vi "Get XPath Text.vi"(8 "error in (no error)":errorcluster, 10 "XPath Expression":string, 11 "DOM document in":refnum<k20>) -> (0 "error out":errorcluster, 1 "Found?":bool, 2 "Node Text":string, 3 "DOM document out":refnum<k20>)   [LabVIEW 2016, in "SLL File IO.lvlib"]
doc: "For the given XPath expression, it returns the node text."
uses:
  SLL File IO.lvlib
  <vilib>/xml/Close Reference(Node).vi
  <vilib>/xml/NI_XML.lvlib
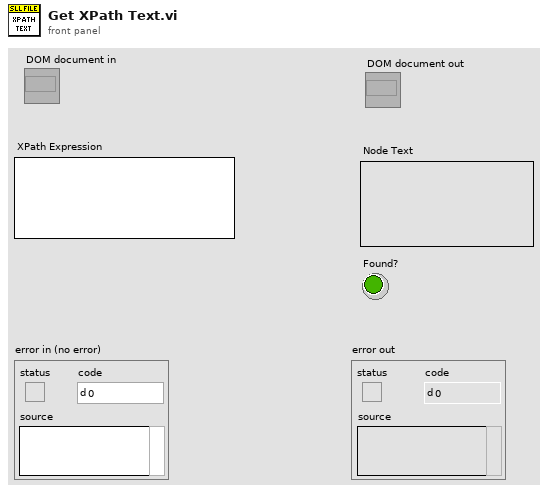
[diagram p1: front panel]
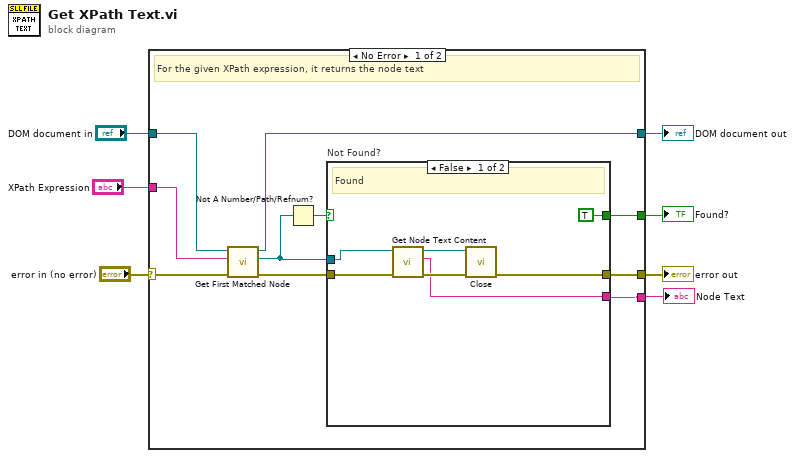
[diagram p0: block diagram]
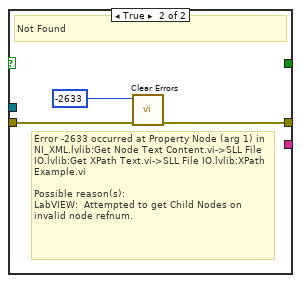
[diagram p2: hidden frame]
diagram:
  n1 = case shown="No Error" "error in (no error)" {
    selector: "error in (no error)" -> [w17 w29]
    tunnel: [w13 w29] -> w6
    tunnel: "XPath Expression" -> [w15 _]
    tunnel: "DOM document in" -> [w14 w28]
    tunnel: [w12 _] -> w3
    tunnel: [w11 w28] -> w2
    tunnel: [w8 _] -> w1
    frame No Error {
      # "For the given XPath expression, it returns the node text"
      n2 = call <vilib>:"Get First Matched Node.vi"("error in (no error)"=w17, "XPath expression"=w15, "node in"=w14) -> ("error out"=w16:errorcluster, "node result"=w10:refnum<k20>, "node out"=w11:refnum<k20>)  [unwired: 6 in]
      n3 = Not A Number/Path/Refnum?(number/path/refnum=w10) -> (NaN/Path/Refnum?=w9:bool)
      n4 = case "Not Found?" shown="False" w9 {
        tunnel: w16 -> [w24 w27]
        tunnel: [w22 w26] -> w13
        tunnel: [w20 _] -> w12
        tunnel: w10 -> [w19 _]
        tunnel: [TRUE _] -> w8
        frame False {
          # "Found"
          n5 = call <vilib>:"Get Node Text Content.vi"("error in (no error)"=w24, "node in"=w19) -> ("error out"=w23:errorcluster, "node text"=w20:string, "node out"=w21:refnum<k20>)  [unwired: 7 in]
          n6 = call-poly <vilib>:"Close.vi"("error in (no error)"=w23, "node"=w21) -> ("error out"=w22:errorcluster)  [unwired: 7 in]
        }
        frame True {
          # "Error -2633 occurred at Property Node (arg 1) in NI_XML.lvlib:Get Node Text Content.vi->SLL File IO.lvlib:Get XPath Text.vi->SLL File IO.lvlib:XPath Example.vi\n\nPossible reason(s):\nLabVIEW:  Attempted to get Child Nodes on invalid node refnum."
          # "Not Found"
          n7 = call <vilib>:"Clear Errors.vi"("error in (no error)"=w27, "specific error code to clear (0: all)"=-2633) -> ("error out"=w26:errorcluster)  [unwired: 4 in, 1 out]
        }
      }
    }
    frame Error {
    }
  }
  "error out" <- w6
  "Node Text" <- w3
  "DOM document out" <- w2
  "Found?" <- w1
